vi "write_spectra_new_Flash.vi"() -> ()   [LabVIEW 2022 SP3]
uses:
  <vilib>/Utility/file.llb/Read From Spreadsheet File (DBL).vi
panel:
  in  "addition":dbl
  in  "multiplied by":dbl=1.0
  out "second subarray":u8[](array[numeric])
  out "first subarray":u8[](array[numeric])
  out "size of array to write":i32
  out "Array to write":u8[](array[numeric])
  out "Waveform Graph 2":u16[](graph)
  in  "first row":dbl[](array[numeric])
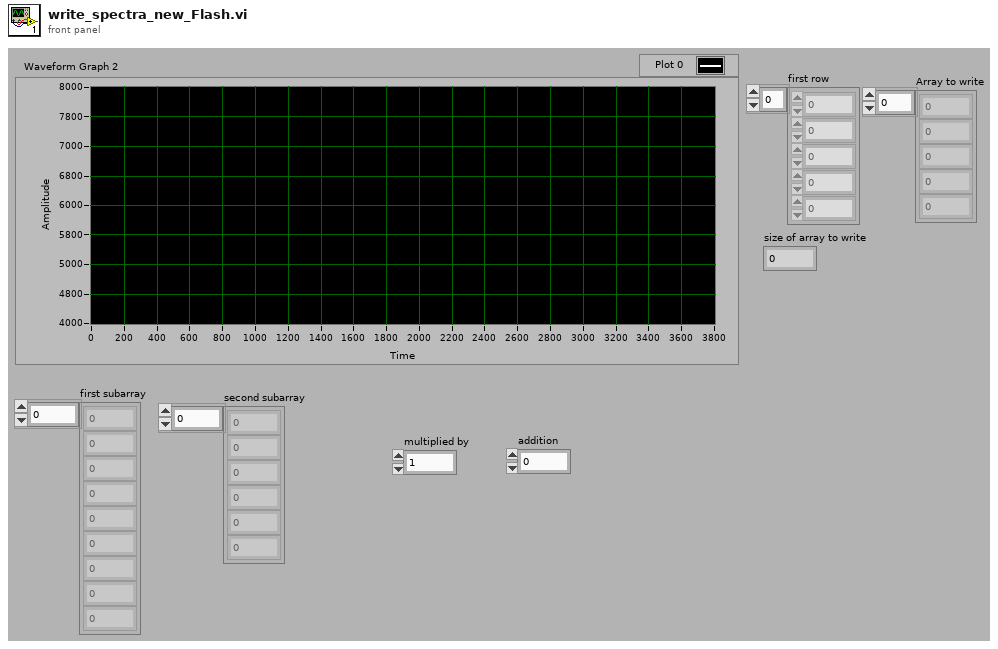
[diagram p1: front panel]
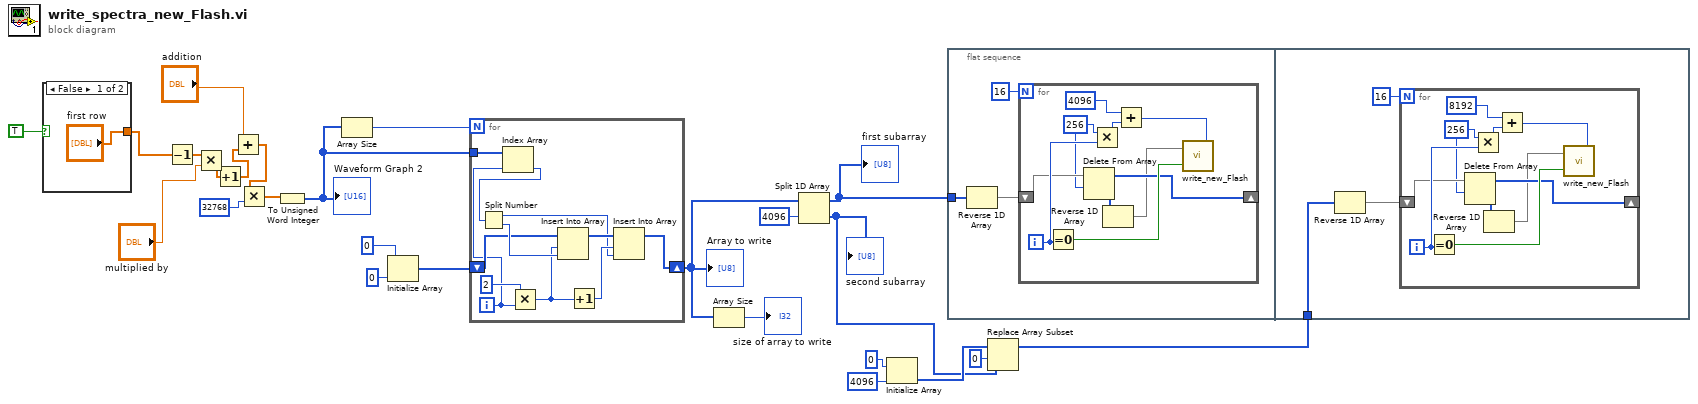
[diagram p0: block diagram]
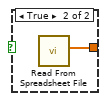
[diagram p2: hidden frame]
diagram:
  n1 = case shown="False" TRUE {
    tunnel: ["first row" w27] -> w7
    frame False {
    }
    frame True {
      n2 = call-poly <vilib>:"Read From Spreadsheet File.vi"() -> ("first row"=w27:dbl[])  [unwired: 7 in, 4 out]
    }
  }
  n3 = Decrement(x=w7) -> (x-1=w6:dbl[])
  n4 = Multiply(x=w6, y="multiplied by") -> (x*y=w5:dbl[])
  n5 = Increment(x=w5) -> (x+1=w3:dbl[])
  n6 = Add(x="addition", y=w3) -> (x+y=w2:dbl[])
  n7 = Multiply(x=w2, y=u16 32768) -> (x*y=w23:dbl[])
  n8 = To Unsigned Word Integer(number=w23) -> (unsigned 16bit integer=w22:u16[])
  "Waveform Graph 2" <- w22
  n9 = Array Size(array=w22) -> (size(s)=w17:i32)
  n10 = Initialize Array(u8 0 ("element"), 0 ("dimension size")) -> (w19:u8[])
  n11 = for {
    N: w17 -> [_]
    tunnel: w22 -> [w30]
    shift-right: [w31] -> w16
    shift-left: w19 -> [w36]
    i -> [w29]
    n12 = Index Array(array=w30, index=w29) -> (element=w28:u16)
    n13 = Split Number(x=w28) -> (hi(x)=w32:u8, lo(x)=w37:u8)
    n14 = Multiply(x=2, y=w29) -> (x*y=w34:i32)
    n15 = Insert Into Array(array=w36, index=w34, new element=w37) -> (w35:u8[])
    n16 = Increment(x=w34) -> (x+1=w33:i32)
    n17 = Insert Into Array(array=w35, index=w33, new element=w32) -> (w31:u8[])
  }
  "Array to write" <- w16
  n18 = Array Size(array=w16) -> (size(s)=→"size of array to write":i32)
  n19 = Split 1D Array(array=w16, index=4096) -> (first subarray=w14:u8[], second subarray=w10:u8[])
  "first subarray" <- w14
  "second subarray" <- w10
  n20 = Initialize Array(u8 0 ("element"), 4096 ("dimension size")) -> (w11:u8[])
  n21 = flat-sequence {
    tunnel: w14 -> [w40]
    tunnel: w9 -> [w52]
    frame #0 {
      n22 = Reverse 1D Array(array=w40) -> (reversed array=w39:u8[])
      n23 = for {
        N: 16 -> [_]
        shift-right: [w44] -> _
        shift-left: w39 -> [w47]
        i -> [w48]
        w46 = 256
        n24 = Equal To 0?(x=w48) -> (x = 0?=w51:bool)
        n25 = Delete From Array(array=w47, length=w46) -> (deleted portion=w43:u8[], array with subset deleted=w44:u8[])  [unwired: 1 in]
        n26 = Multiply(x=w46, y=w48) -> (x*y=w45:i32)
        n27 = Reverse 1D Array(array=w43) -> (reversed array=w42:u8[])
        n28 = Add(x=4096, y=w45) -> (x+y=w49:i32)
        n29 = call "write_new_Flash.vi"("address (3 bytes)"=w49, "sector erase"=w51, "write array"=w42) -> ()
      }
    }
    frame #1 {
      n30 = Reverse 1D Array(array=w52) -> (reversed array=w54:u8[])
      n31 = for {
        N: 16 -> [_]
        shift-right: [w57] -> _
        shift-left: w54 -> [w60]
        i -> [w61]
        w59 = 256
        n32 = Equal To 0?(x=w61) -> (x = 0?=w64:bool)
        n33 = Delete From Array(array=w60, length=w59) -> (deleted portion=w56:u8[], array with subset deleted=w57:u8[])  [unwired: 1 in]
        n34 = Multiply(x=w59, y=w61) -> (x*y=w58:i32)
        n35 = Reverse 1D Array(array=w56) -> (reversed array=w55:u8[])
        n36 = Add(x=8192, y=w58) -> (x+y=w62:i32)
        n37 = call "write_new_Flash.vi"("address (3 bytes)"=w62, "sector erase"=w64, "write array"=w55) -> ()
      }
    }
  }
  n38 = Replace Array Subset(array=w11, new element=w10, index=0) -> (w9:u8[])
